vi "ExtTrigAuger clocked option unfinished.vi"() -> ()   [LabVIEW 2014]
uses:
  FPGA state.ctl
  <vilib>/Platform/TimedLoop/XDataNode/timing_clust.ctl
  <vilib>/Platform/TimedLoop/XDataNode/nitl_modes.ctl
  <vilib>/Platform/TimedLoop/XDataNode/wakeup.ctl
  <vilib>/rvi/Emulation/niFpgaSctlEmulationGetInTimedLoop.vi
  <vilib>/rvi/Emulation/niFpgaEmulationReportErrorSimple.vi
  <vilib>/rvi/Emulation/niFpgaGetClockAttributes.vi
  <vilib>/rvi/Emulation/niFpgaCriticalErrorInLSC.vi
  <vilib>/rvi/eio/common/nirviEmuTemplateMethod_errors.vi
  <vilib>/rvi/interface/RandomDataEmulation/niFpgaRandomDataHandleErrors.vi
  <vilib>/Platform/TimedLoop/XDataNode/XDataNode.xnode
  <vilib>/eio/EIONode/EIONode.xnode
  <vilib>/rvi/DataTransferAndStorage/Container/XNode/niFpgaContainer.xnode
  <vilib>/rvi/interface/RandomDataEmulation/nirviRandomDataFpgaReadWriteTemplate.vi
  <vilib>/Platform/TimedLoop/XDataNode/XDNodeRunTimeDep.lvlib
panel:
  in  "Clocked Tick Count":u32=25
  in  "Clocked Sample Count":u32
  out "Overflow":bool
  in  "Trigger Mode":T1(ring)
  # "Each U64 FIFO element is a pair of U32 with\n28 bits data, 4 bit ID in msb\n\nOn trigger or clock timeout\nreturn sample count, delta T in first element,\nand counts since last trigger on the eight data channels\n(7 for Auger plus aux) in the next 4 elements\n\nOn overflow, set trigger mode to off and flush FIFO\nOFF mode clears overflow, also resests sample count"
  # "ExtTrig AugerCounter"
  # "Acquisition can be controlled by external trigger\n(through PXI backplane or input connector)\nor by the FPGA 25 MHz Clock. After sample count\nis reached in clocked mode, trigger mode goes to off\nIf sample count is zero, clocked mode runs forever"
  # "FPGA DMA-FIFO CANNOT be cleared by FPGA,\nonly by PC Host VI. Ctr Overflow will be on when\nFPGA-side FIFO is full!"
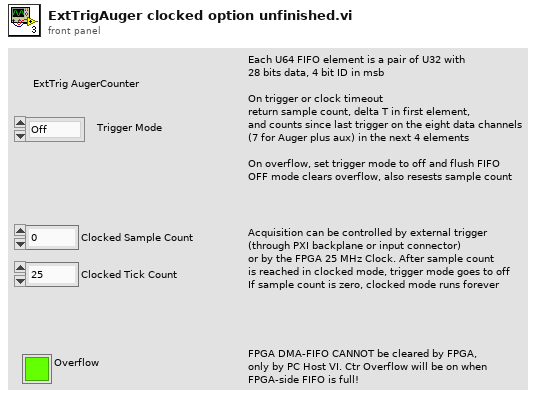
[diagram p1: front panel]
types:
  T1 = enum16{"Off", "PXI Trig0", "DIO-08 Trig", "Clocked"}
  T2 = typedef "FPGA state.ctl" = enum8{"Wait", "Triggered", "Transfer 1", "Transfer 2", "Transfer 3", "Transfer 4", "Overflow"}
  T3 = typedef "XDNodeRunTimeDep.lvlib/timing_clust.ctl" = cluster{"Expected End [f-1]":u64, "Actual End [f-1]":u64, "Finished Late? [f-1]":bool, "Expected End [i-1]":u64, "Actual End [i-1]":u64, "Finished Late? [i-1]":bool, "Expected Start [i]":u64, "Actual Start [i]":u64, "Expected Start [f]":u64, "Actual Start [f]":u64, "Source Name":string, "Structure Name":string, "Period":i64, "Deadline":i64, "Offset":i64, "Start":i64, "Priority":i32, "Timeout":i32, "Mode":T4, "Wakeup Reason":T5, "Error":errorcluster, "Source Type":string, "Secondary Source Type":string, "Global End Time":u64, "Global Start Time":u64, "Frame Duration":u64, "Iteration Duration":u64, "Assigned CPU":i32, "I/O Scan Engine Mode":u32}
  T4 = typedef "XDNodeRunTimeDep.lvlib/nitl_modes.ctl" = enum32{"No Change", "Process missed periods, maintain original phase", "Discard missed periods, maintain original phase", "Process missed periods, ignore original phase", "Discard missed periods, ignore original phase"}
  T5 = typedef "XDNodeRunTimeDep.lvlib/wakeup.ctl" = enum32{"Normal", "Aborted", "Asynchronous wakeup", "Timing source error", "Timed loop error", "Timeout"}
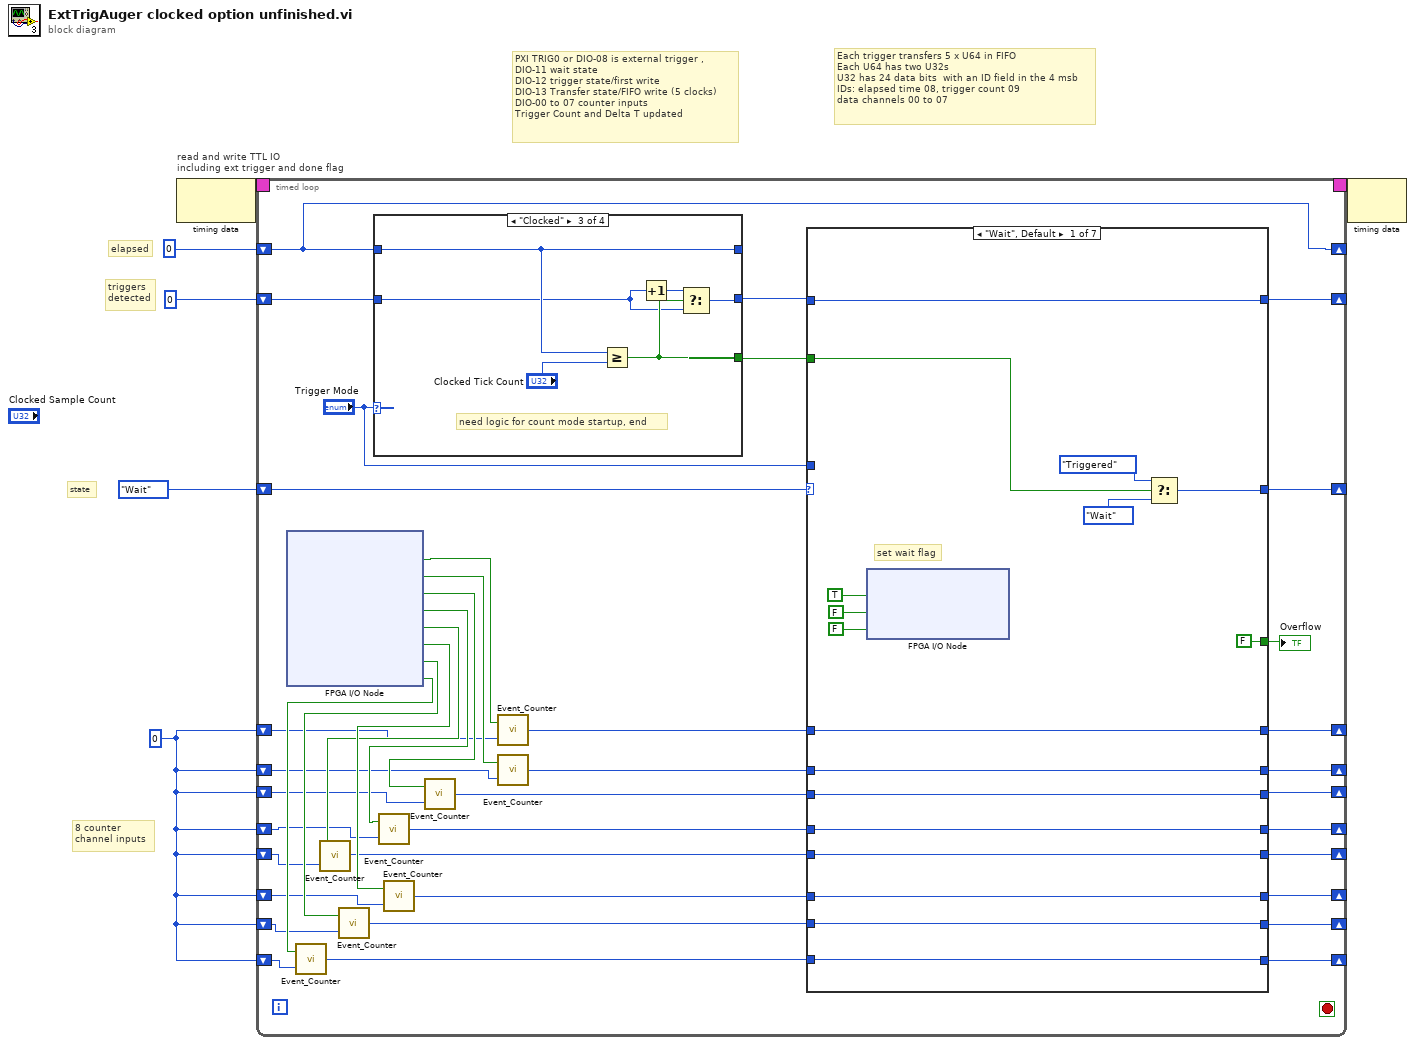
[diagram p0: block diagram]
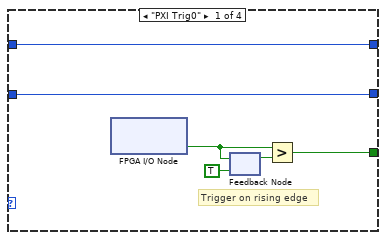
[diagram p2: hidden frame]
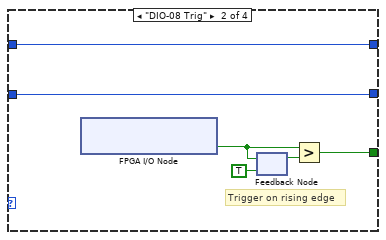
[diagram p3: hidden frame]
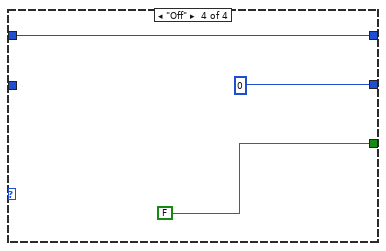
[diagram p4: hidden frame]
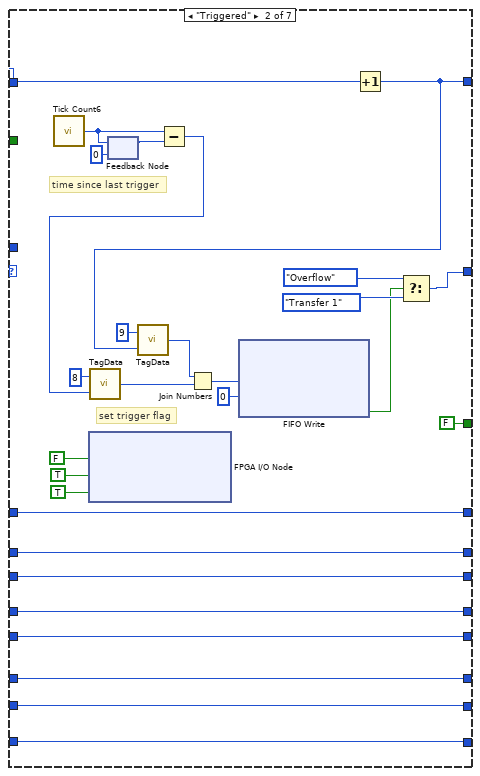
[diagram p5: hidden frame]
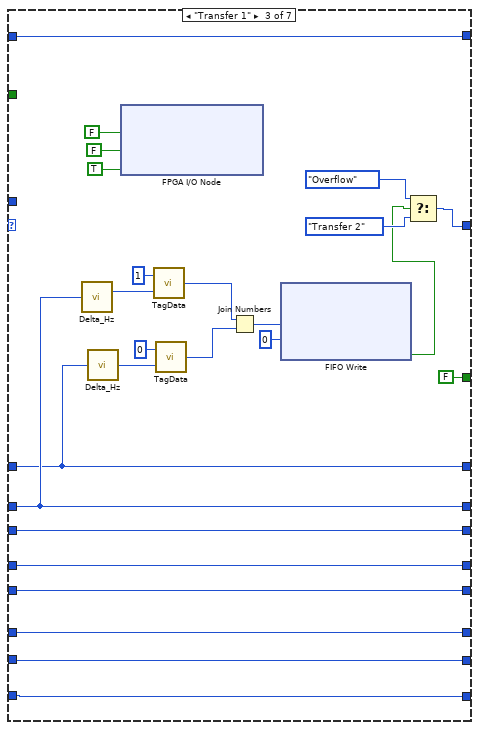
[diagram p6: hidden frame]
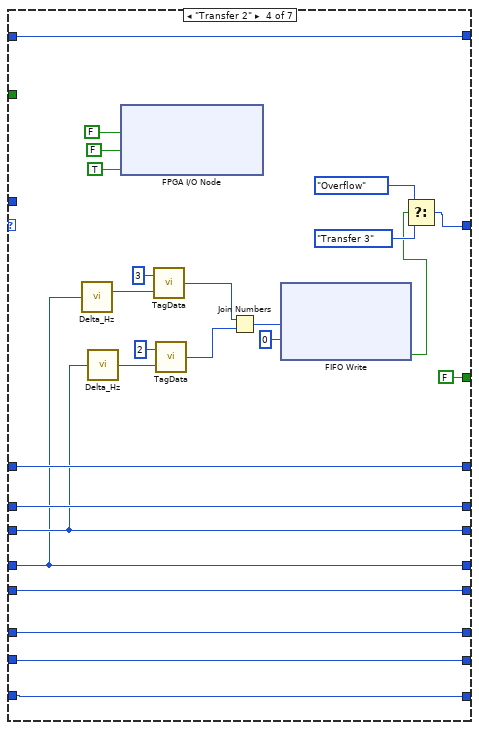
[diagram p7: hidden frame]
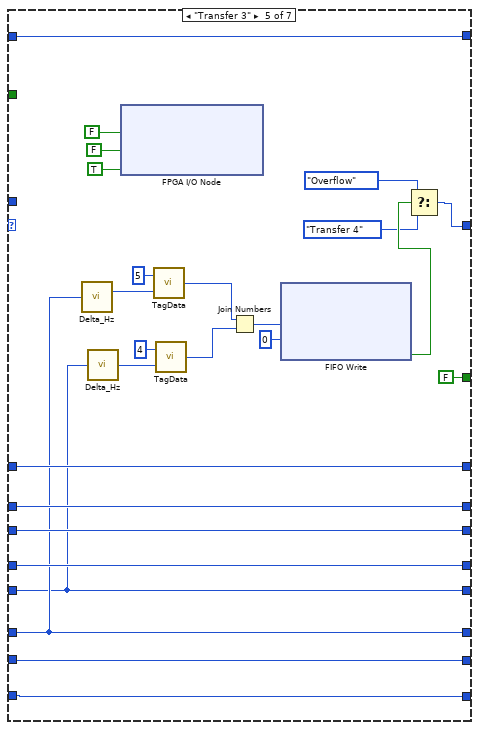
[diagram p8: hidden frame]
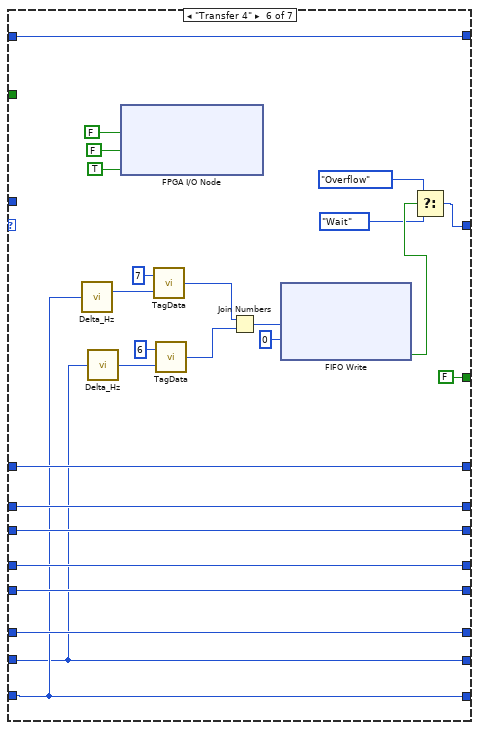
[diagram p9: hidden frame]
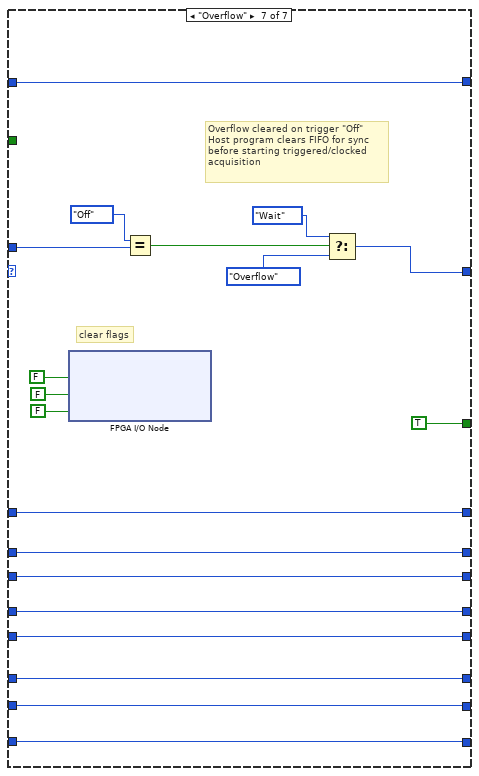
[diagram p10: hidden frame]
diagram:
  w1 = u32 0 ("Counts out")
  # "Each trigger transfers 5 x U64 in FIFO\nEach U64 has two U32s\nU32 has 24 data bits  with an ID field in the 4 msb\nIDs: elapsed time 08, trigger count 09\ndata channels 00 to 07"
  # "8 counter\nchannel inputs"
  # "elapsed"
  # "state"
  # "triggers\ndetected"
  # "PXI TRIG0 or DIO-08 is external trigger ,\nDIO-11 wait state\nDIO-12 trigger state/first write \nDIO-13 Transfer state/FIFO write (5 clocks)\nDIO-00 to 07 counter inputs \nTrigger Count and Delta T updated"
  n1 = node-c288() -> (w6:T3)  [unwired: 1 in]
  n2 = timed-loop "read and write TTL IO\nincluding ext trigger and done flag" {
    timing: w6 -> [_]
    timing-out: [_] -> w5
    shift-right: [w46] -> _
    shift-left: FPGA_state."Wait" -> [w47]
    shift-right: [w45] -> _
    shift-left: u32 0 -> [w11]
    shift-right: [w7] -> _
    shift-left: u32 0 -> [w7]
    shift-right: [w13] -> _
    shift-left: w1 -> [w29]
    shift-right: [w16] -> _
    shift-left: w1 -> [w30]
    shift-right: [w15] -> _
    shift-left: w1 -> [w34]
    shift-right: [w19] -> _
    shift-left: w1 -> [w35]
    shift-right: [w22] -> _
    shift-left: w1 -> [w38]
    shift-right: [w23] -> _
    shift-left: w1 -> [w37]
    shift-right: [w26] -> _
    shift-left: w1 -> [w39]
    shift-right: [w27] -> _
    shift-left: w1 -> [w40]
    stop <- _ stop-if-true
    n3 = xnode "FPGA I/O Node"() -> ("Connector0/DIO0"=w31:bool, "Connector0/DIO1"=w32:bool, "Connector0/DIO2"=w33:bool, "Connector0/DIO3"=w36:bool, "Connector0/DIO4"=w41:bool, "Connector0/DIO5"=w42:bool, "Connector0/DIO6"=w43:bool, "Connector0/DIO7"=w44:bool)  [unwired: 8 in, 8 out]
    n4 = call "Event_Counter.vi"("Counts in"=w40, "input"=w44) -> ("Counts out"=w28:u32)
    n5 = call "Event_Counter.vi"("Counts in"=w38, "input"=w41) -> ("Counts out"=w21:u32)
    n6 = call "Event_Counter.vi"("Counts in"=w39, "input"=w43) -> ("Counts out"=w25:u32)
    n7 = case shown="\"Clocked\"" "Trigger Mode" {
      tunnel: [w49 w56 w63 FALSE ("Connector0/DIO8")] -> w8
      tunnel: w11 -> [w53 w59 w61 _]
      tunnel: [w53 w59 w60 u32 0] -> w9
      tunnel: w7 -> [w48 w54 w64 w66]
      tunnel: [w48 w54 w64 w66] -> _
      frame "PXI Trig0" {
        # "Trigger on rising edge"
        n8 = xnode "FPGA I/O Node"() -> ("TRIG0"=w50:bool)  [unwired: 1 in, 1 out]
        n9 = feedback #1(TRUE ("set")) -> (w51:bool)
        n10 = feedback-in #1(w50) -> ()
        n11 = Greater?(x=w50, y=w51) -> (0:w49:bool)
      }
      frame "DIO-08 Trig" {
        # "Trigger on rising edge"
        n12 = xnode "FPGA I/O Node"() -> ("Connector0/DIO8"=w55:bool)  [unwired: 1 in, 1 out]
        n13 = feedback #2(TRUE ("set")) -> (w58:bool)
        n14 = feedback-in #2(w55) -> ()
        n15 = Greater?(x=w55, y=w58) -> (0:w56:bool)
      }
      frame "Clocked" {
        # "need logic for count mode startup, end"
        n16 = Greater Or Equal?(x=w64, y="Clocked Tick Count") -> (x >= y?=w63:bool)
        n17 = Increment(x=w61) -> (x+1=w62:u32)
        n18 = Select(t=w62, s=w63, f=w61) -> (s? t:f=w60:u32)
      }
      frame "Off" {
      }
    }
    n19 = call "Event_Counter.vi"("Counts in"=w35, "input"=w36) -> ("Counts out"=w20:u32)
    n20 = call "Event_Counter.vi"("Counts in"=w37, "input"=w42) -> ("Counts out"=w24:u32)
    n21 = call "Event_Counter.vi"("Counts in"=w34, "input"=w33) -> ("Counts out"=w18:u32)
    n22 = call "Event_Counter.vi"("Counts in"=w29, "input"=w31) -> ("Counts out"=w14:u32)
    n23 = call "Event_Counter.vi"("Counts in"=w30, "input"=w32) -> ("Counts out"=w17:u32)
    n24 = case shown="\"Wait\", Default" w47 {
      tunnel: [w83 w91 w115 w140 w165 w190 w214] -> w46
      tunnel: w9 -> [w81 w113 w131 w156 w181 w206 w232]
      tunnel: [w81 w92 w131 w156 w181 w206 w232] -> w45
      tunnel: w8 -> [w82 _ _ _ _ _ _]
      tunnel: w28 -> [w80 w106 w124 w150 w177 w195 w231]
      tunnel: [w80 w106 w124 w150 w177 w195 w231] -> w27
      tunnel: [w79 w105 w125 w151 w178 w194 w230] -> w26
      tunnel: w25 -> [w79 w105 w125 w151 w178 w194 w230]
      tunnel: w24 -> [w78 w104 w126 w152 w170 w197 w229]
      tunnel: [w78 w104 w126 w152 w170 w197 w229] -> w23
      tunnel: [w77 w103 w127 w153 w169 w196 w228] -> w22
      tunnel: w21 -> [w77 w103 w127 w153 w169 w196 w228]
      tunnel: w20 -> [w76 w99 w123 w144 w171 w198 w227]
      tunnel: [w76 w99 w123 w144 w171 w198 w227] -> w19
      tunnel: w18 -> [w74 w102 w128 w145 w172 w199 w225]
      tunnel: w17 -> [w75 w101 w120 w147 w174 w201 w226]
      tunnel: [w75 w101 w120 w147 w174 w201 w226] -> w16
      tunnel: [w74 w102 w128 w145 w172 w199 w225] -> w15
      tunnel: w14 -> [w73 w100 w119 w146 w173 w200 w224]
      tunnel: [w73 w100 w119 w146 w173 w200 w224] -> w13
      tunnel: [FALSE ("Connector0/DIO11") FALSE ("Connector0/DIO11") FALSE ("Connector0/DIO11") FALSE ("Connector0/DIO11") FALSE ("Connector0/DIO11") FALSE ("Connector0/DIO11") TRUE ("Connector0/DIO11")] -> w12
      tunnel: "Trigger Mode" -> [_ _ _ _ _ _ w219]
      frame "Wait", Default {
        # "set wait flag"
        n25 = xnode "FPGA I/O Node"("Connector0/DIO11"=TRUE, "Connector0/DIO12"=FALSE ("Connector0/DIO11"), "Connector0/DIO13"=FALSE ("Connector0/DIO11")) -> ()  [unwired: 3 in, 3 out]
        n26 = Select(t=FPGA_state."Triggered", s=w82, f=FPGA_state."Wait") -> (s? t:f=w83:T2)
      }
      frame "Triggered" {
        # "time since last trigger"
        # "set trigger flag"
        n27 = Increment(x=w113) -> ()  [unwired: 1 out]
        n28 = call "Tick Count6"() -> ("Tick Count(Ticks)"=w111:u32)
        n29 = xnode "FPGA I/O Node"("Connector0/DIO11"=FALSE, "Connector0/DIO12"=TRUE ("Connector0/DIO11"), "Connector0/DIO13"=TRUE ("Connector0/DIO11")) -> ()  [unwired: 3 in, 3 out]
        n30 = feedback-in #3(w111) -> ()
        n31 = feedback #3(u32 0 ("Tick Count(Ticks)")) -> (w112:u32)
        n32 = Subtract(x=w111, y=w112) -> (x-y=w86:u32)
        n33 = call "TagData.vi"("Data"=w86, "Tag"=u8 8) -> ("Data 2"=w93:u32)
        n34 = Increment(x=w113) -> (x+1=w92:u32)
        n35 = call "TagData.vi"("Data"=w92, "Tag"=u8 9) -> ("Data 2"=w96:u32)
        n36 = Join Numbers(hi=w96, lo=w93) -> ((hi.lo)=w98:u64)
        n37 = xnode ("FIFO Write")("Element"=w98, "Timeout"=0) -> ("Timed Out?"=w88:bool)  [unwired: 1 in, 1 out]
        n38 = Select(t=FPGA_state."Overflow", s=w88, f=FPGA_state."Transfer 1") -> (s? t:f=w91:T2)
      }
      frame "Transfer 1" {
        n39 = call "Delta_Hz.vi"("Counts"=w120) -> ("Delta"=w121:u32)
        n40 = call "Delta_Hz.vi"("Counts"=w119) -> ("Delta"=w122:u32)
        n41 = xnode "FPGA I/O Node"("Connector0/DIO11"=FALSE ("Connector0/DIO15"), "Connector0/DIO12"=FALSE ("Connector0/DIO15"), "Connector0/DIO13"=TRUE ("Connector0/DIO15")) -> ()  [unwired: 3 in, 3 out]
        n42 = call "TagData.vi"("Data"=w121, "Tag"=u8 1) -> ("Data 2"=w133:u32)
        n43 = call "TagData.vi"("Data"=w122, "Tag"=u8 0) -> ("Data 2"=w129:u32)
        n44 = Join Numbers(hi=w133, lo=w129) -> ((hi.lo)=w138:u64)
        n45 = xnode ("FIFO Write")("Element"=w138, "Timeout"=0) -> ("Timed Out?"=w116:bool)  [unwired: 1 in, 1 out]
        n46 = Select(t=FPGA_state."Overflow", s=w116, f=FPGA_state."Transfer 2") -> (s? t:f=w115:T2)
      }
      frame "Transfer 2" {
        n47 = call "Delta_Hz.vi"("Counts"=w144) -> ("Delta"=w148:u32)
        n48 = call "Delta_Hz.vi"("Counts"=w145) -> ("Delta"=w149:u32)
        n49 = xnode "FPGA I/O Node"("Connector0/DIO11"=FALSE ("Connector0/DIO15"), "Connector0/DIO12"=FALSE ("Connector0/DIO15"), "Connector0/DIO13"=TRUE ("Connector0/DIO15")) -> ()  [unwired: 3 in, 3 out]
        n50 = call "TagData.vi"("Data"=w148, "Tag"=u8 3) -> ("Data 2"=w158:u32)
        n51 = call "TagData.vi"("Data"=w149, "Tag"=u8 2) -> ("Data 2"=w154:u32)
        n52 = Join Numbers(hi=w158, lo=w154) -> ((hi.lo)=w163:u64)
        n53 = xnode ("FIFO Write")("Element"=w163, "Timeout"=0) -> ("Timed Out?"=w142:bool)  [unwired: 1 in, 1 out]
        n54 = Select(t=FPGA_state."Overflow", s=w142, f=FPGA_state."Transfer 3") -> (s? t:f=w140:T2)
      }
      frame "Transfer 3" {
        n55 = call "Delta_Hz.vi"("Counts"=w170) -> ("Delta"=w175:u32)
        n56 = call "Delta_Hz.vi"("Counts"=w169) -> ("Delta"=w176:u32)
        n57 = xnode "FPGA I/O Node"("Connector0/DIO11"=FALSE ("Connector0/DIO15"), "Connector0/DIO12"=FALSE ("Connector0/DIO15"), "Connector0/DIO13"=TRUE ("Connector0/DIO15")) -> ()  [unwired: 3 in, 3 out]
        n58 = call "TagData.vi"("Data"=w175, "Tag"=u8 5) -> ("Data 2"=w183:u32)
        n59 = call "TagData.vi"("Data"=w176, "Tag"=u8 4) -> ("Data 2"=w179:u32)
        n60 = Join Numbers(hi=w183, lo=w179) -> ((hi.lo)=w188:u64)
        n61 = xnode ("FIFO Write")("Element"=w188, "Timeout"=0) -> ("Timed Out?"=w168:bool)  [unwired: 1 in, 1 out]
        n62 = Select(t=FPGA_state."Overflow", s=w168, f=FPGA_state."Transfer 4") -> (s? t:f=w165:T2)
      }
      frame "Transfer 4" {
        n63 = call "Delta_Hz.vi"("Counts"=w195) -> ("Delta"=w202:u32)
        n64 = call "Delta_Hz.vi"("Counts"=w194) -> ("Delta"=w203:u32)
        n65 = xnode "FPGA I/O Node"("Connector0/DIO11"=FALSE ("Connector0/DIO15"), "Connector0/DIO12"=FALSE ("Connector0/DIO15"), "Connector0/DIO13"=TRUE ("Connector0/DIO15")) -> ()  [unwired: 3 in, 3 out]
        n66 = call "TagData.vi"("Data"=w202, "Tag"=u8 7) -> ("Data 2"=w208:u32)
        n67 = call "TagData.vi"("Data"=w203, "Tag"=u8 6) -> ("Data 2"=w204:u32)
        n68 = Join Numbers(hi=w208, lo=w204) -> ((hi.lo)=w213:u64)
        n69 = xnode ("FIFO Write")("Element"=w213, "Timeout"=0) -> ("Timed Out?"=w193:bool)  [unwired: 1 in, 1 out]
        n70 = Select(t=FPGA_state."Overflow", s=w193, f=FPGA_state."Wait") -> (s? t:f=w190:T2)
      }
      frame "Overflow" {
        # "Overflow cleared on trigger \"Off\"\nHost program clears FIFO for sync\nbefore starting triggered/clocked\nacquisition"
        # "clear flags"
        n71 = xnode "FPGA I/O Node"("Connector0/DIO11"=FALSE, "Connector0/DIO12"=FALSE ("Connector0/DIO11"), "Connector0/DIO13"=FALSE ("Connector0/DIO11")) -> ()  [unwired: 3 in, 3 out]
        n72 = Equal?(x=T1."Off" ("Trigger Mode"), y=w219) -> (x = y?=w217:bool)
        n73 = Select(t=FPGA_state."Wait", s=w217, f=FPGA_state."Overflow") -> (s? t:f=w214:T2)
      }
    }
    "Overflow" <- w12
  }
  n74 = node-c288(w5) -> ()  [unwired: 1 out]
